vi "construct mysql.vi"(8 "error in (no error)":errorcluster, 10 "Connection string":string="server=127.0.0.1;uid=root;pwd=Nitrog3n;database=test") -> (0 "error out":errorcluster, 3 "mysql out":refnum<class "mysql.lvclass">)   [LabVIEW 2020, in "mysql.lvlib" / "mysql.lvclass"]
uses:
  mysql.net/mysql.lvclass
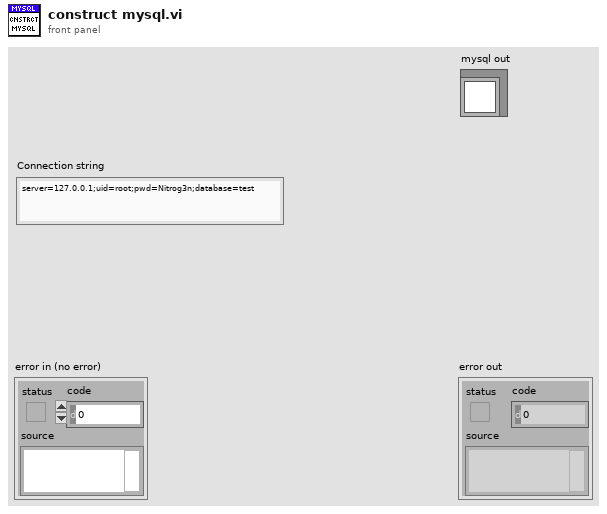
[diagram p1: front panel]
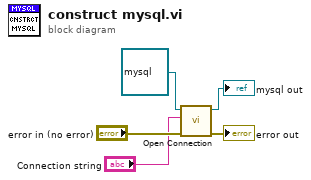
[diagram p0: block diagram]
diagram:
  n1 = call-dynamic "Open Connection.vi"("error in (no error)"="error in (no error)", "Connection string"="Connection string", "mysql in"=refnum<class "mysql.lvclass"> refnum) -> ("error out"=→"error out":errorcluster, "mysql out"=→"mysql out":refnum<class "mysql.lvclass">)  [unwired: 7 in]
